vi "Init6733.vi"(8 "error in":errorcluster caption="错误输入") -> (0 "error out":errorcluster caption="错误输出", 3 "task out":refnum<k21> caption="任务输出")   [LabVIEW 2014]
uses:
  <vilib>/DAQmx/create/channels.llb/DAQmx Create Channel (AO-Voltage-Basic).vi
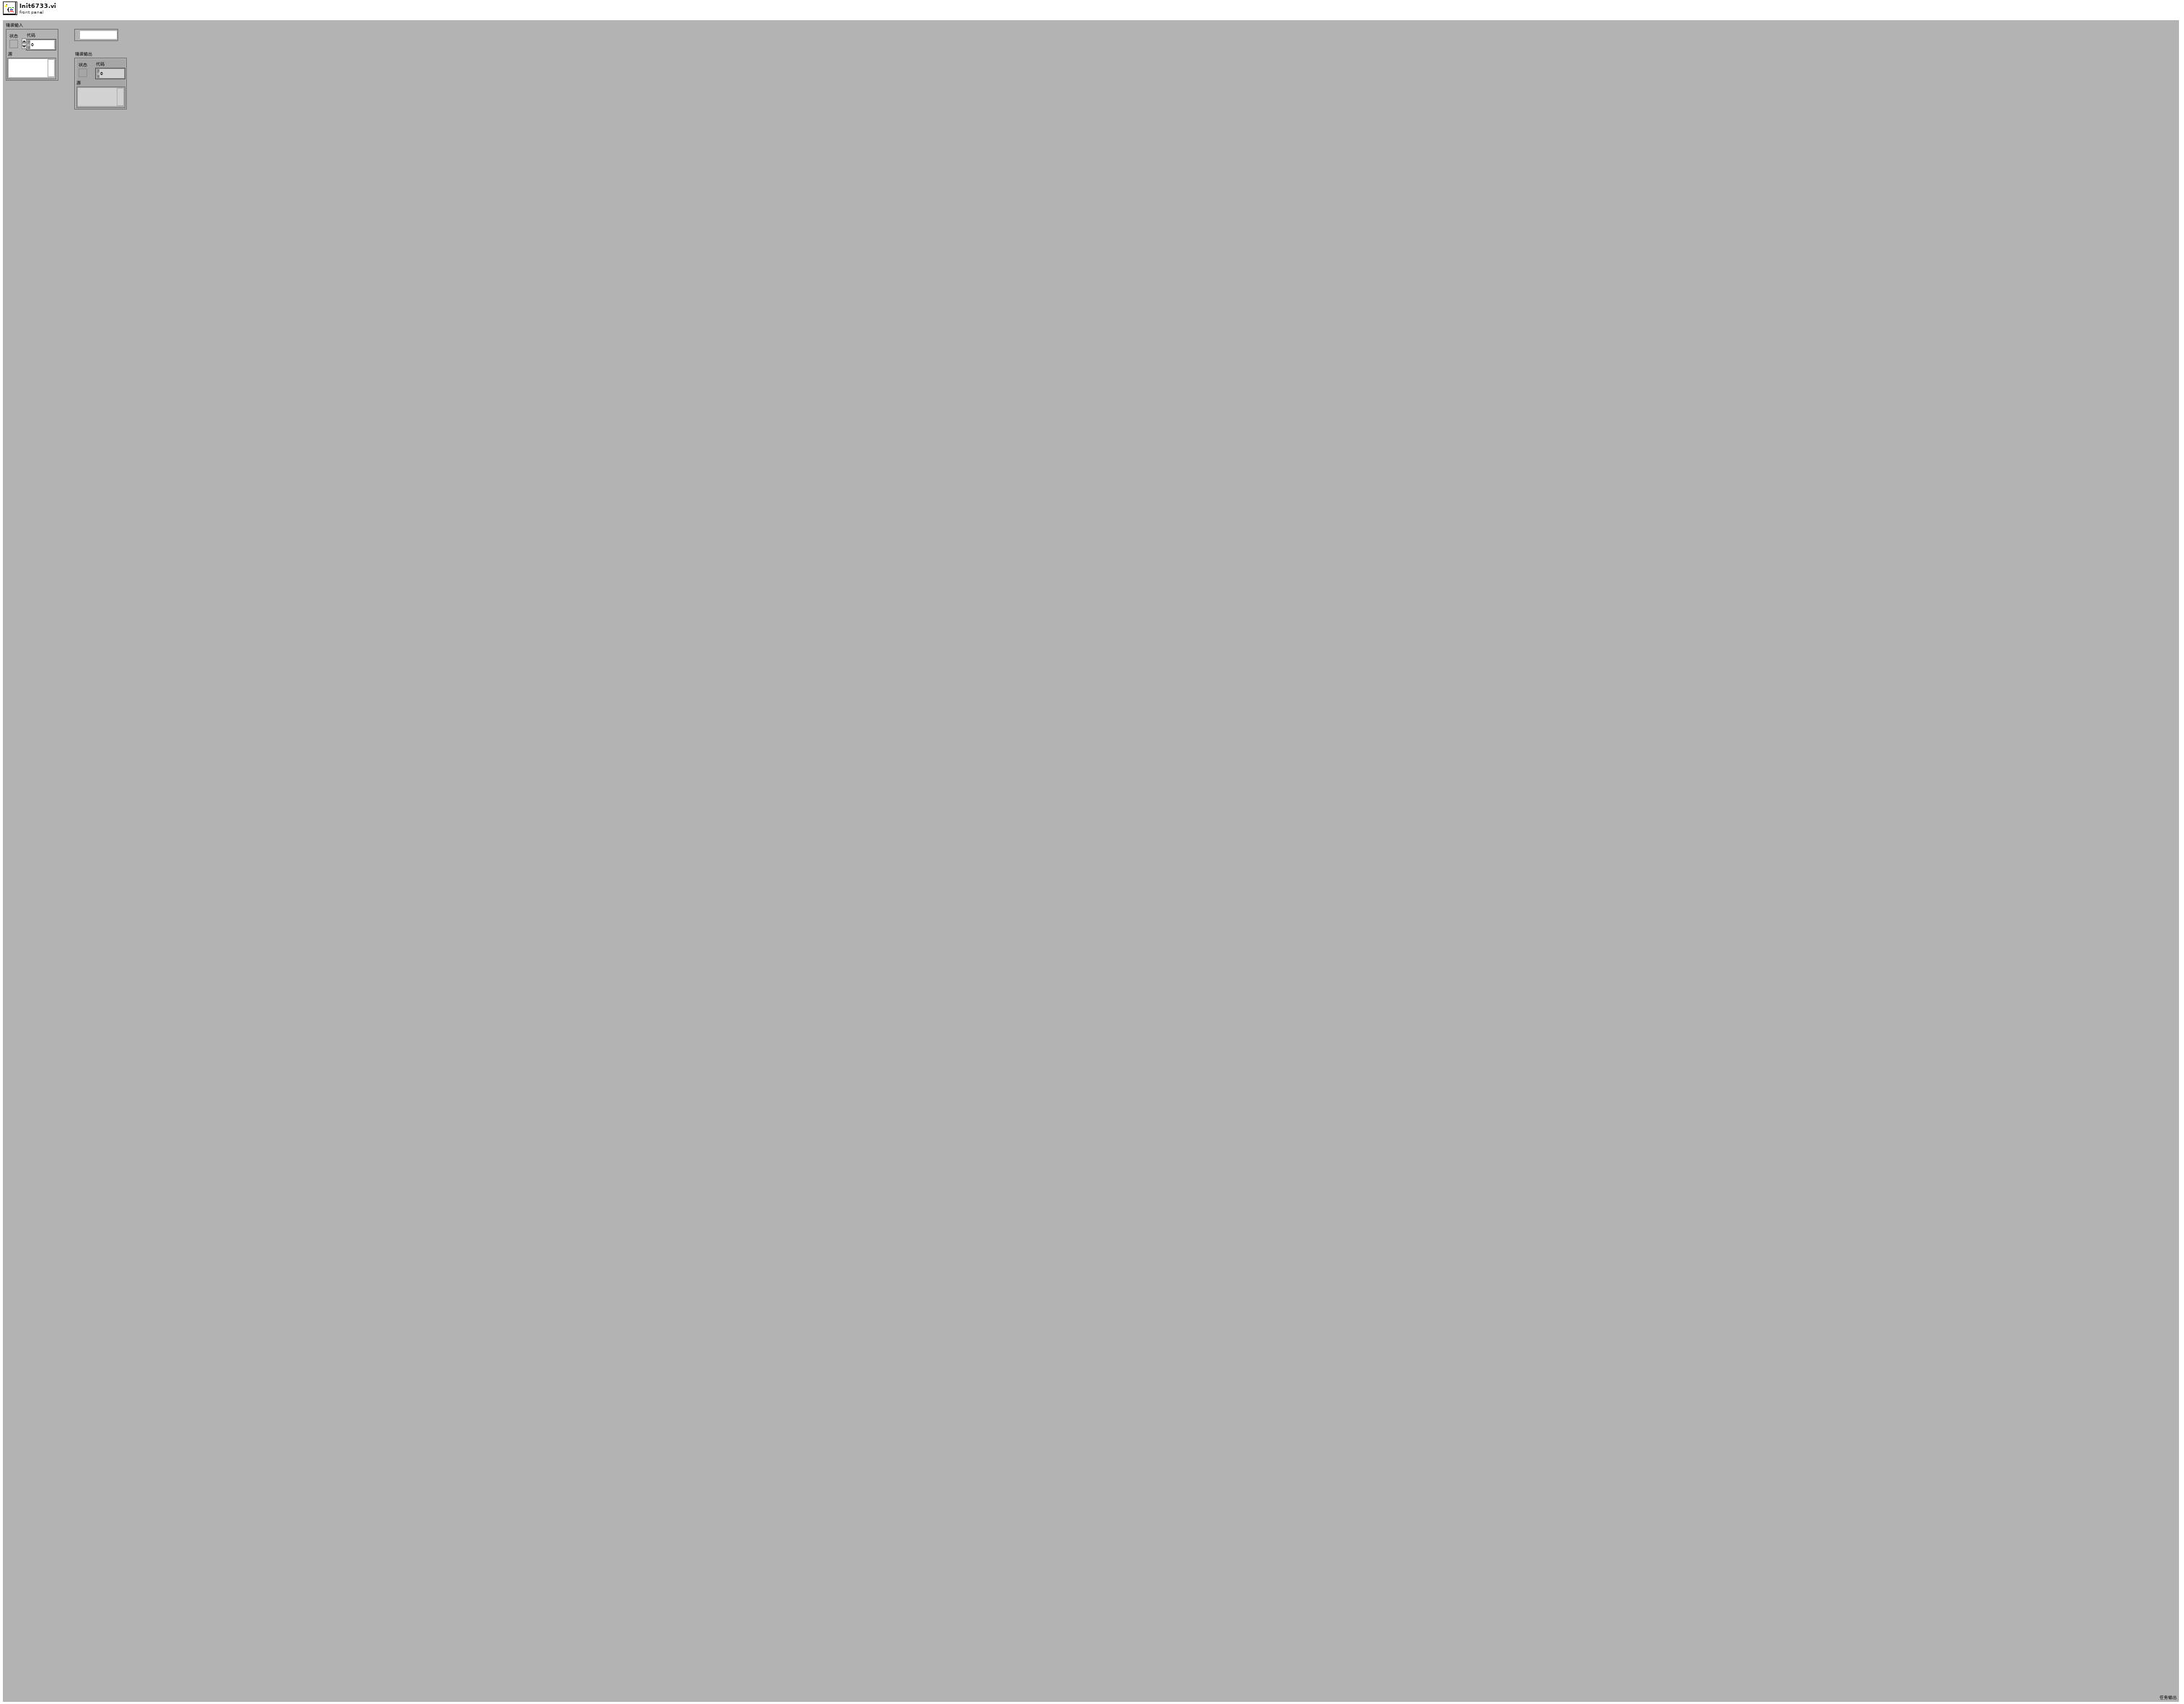
[diagram p1: front panel]
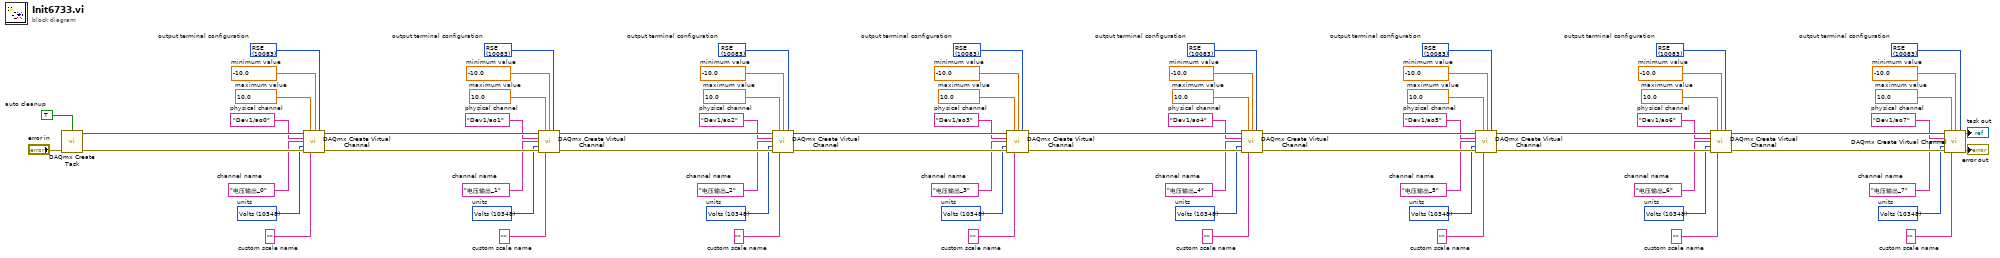
[diagram p0: block diagram]
diagram:
  w1 = 10083 items=["Default"=-1, "RSE"=10083, "Differential"=10106, "Pseudodifferential"=12529]  # output terminal configuration
  w2 = 10348 items=["Volts"=10348, "From Custom Scale"=10065]  # units
  w3 = "电压输出_7"  # channel name
  w6 = ""  # custom scale name
  w7 = -10.0  # minimum value
  w8 = 10.0  # maximum value
  w9 = "Dev1/ao7"  # physical channel
  w11 = 10083 items=["Default"=-1, "RSE"=10083, "Differential"=10106, "Pseudodifferential"=12529]  # output terminal configuration
  w12 = 10348 items=["Volts"=10348, "From Custom Scale"=10065]  # units
  w13 = "电压输出_6"  # channel name
  w15 = ""  # custom scale name
  w16 = -10.0  # minimum value
  w17 = 10.0  # maximum value
  w18 = "Dev1/ao6"  # physical channel
  w20 = 10083 items=["Default"=-1, "RSE"=10083, "Differential"=10106, "Pseudodifferential"=12529]  # output terminal configuration
  w21 = 10348 items=["Volts"=10348, "From Custom Scale"=10065]  # units
  w22 = "电压输出_5"  # channel name
  w24 = ""  # custom scale name
  w25 = -10.0  # minimum value
  w26 = 10.0  # maximum value
  w27 = "Dev1/ao5"  # physical channel
  w29 = 10083 items=["Default"=-1, "RSE"=10083, "Differential"=10106, "Pseudodifferential"=12529]  # output terminal configuration
  w30 = 10348 items=["Volts"=10348, "From Custom Scale"=10065]  # units
  w31 = "电压输出_4"  # channel name
  w33 = ""  # custom scale name
  w34 = -10.0  # minimum value
  w35 = 10.0  # maximum value
  w36 = "Dev1/ao4"  # physical channel
  w38 = 10083 items=["Default"=-1, "RSE"=10083, "Differential"=10106, "Pseudodifferential"=12529]  # output terminal configuration
  w39 = 10348 items=["Volts"=10348, "From Custom Scale"=10065]  # units
  w40 = "电压输出_3"  # channel name
  w42 = ""  # custom scale name
  w43 = -10.0  # minimum value
  w44 = 10.0  # maximum value
  w45 = "Dev1/ao3"  # physical channel
  w47 = 10083 items=["Default"=-1, "RSE"=10083, "Differential"=10106, "Pseudodifferential"=12529]  # output terminal configuration
  w48 = 10348 items=["Volts"=10348, "From Custom Scale"=10065]  # units
  w49 = "电压输出_2"  # channel name
  w51 = ""  # custom scale name
  w52 = -10.0  # minimum value
  w53 = 10.0  # maximum value
  w54 = "Dev1/ao2"  # physical channel
  w56 = 10083 items=["Default"=-1, "RSE"=10083, "Differential"=10106, "Pseudodifferential"=12529]  # output terminal configuration
  w57 = 10348 items=["Volts"=10348, "From Custom Scale"=10065]  # units
  w58 = "电压输出_1"  # channel name
  w60 = ""  # custom scale name
  w61 = -10.0  # minimum value
  w62 = 10.0  # maximum value
  w63 = "Dev1/ao1"  # physical channel
  w65 = 10083 items=["Default"=-1, "RSE"=10083, "Differential"=10106, "Pseudodifferential"=12529]  # output terminal configuration
  w66 = 10348 items=["Volts"=10348, "From Custom Scale"=10065]  # units
  w67 = "电压输出_0"  # channel name
  w69 = ""  # custom scale name
  w70 = -10.0  # minimum value
  w71 = 10.0  # maximum value
  w72 = "Dev1/ao0"  # physical channel
  w74 = TRUE  # auto cleanup
  n1 = call <vilib>:"DAQmx Create Task.vi"("auto cleanup"=w74, "error in"="error in") -> ("task out"=w73:refnum<k21>, "error out"=w75:errorcluster)  [unwired: 12 in]
  n2 = call-poly <vilib>:"DAQmx Create Virtual Channel.vi"("task in"=w73, "maximum value"=w71, "minimum value"=w70, "output terminal configuration"=w65, "physical channels"=w72, "name to assign"=w67, "units"=w66, "error in"=w75, "custom scale name"=w69) -> ("task out"=w64:refnum<k21>, "error out"=w68:errorcluster)  [unwired: 5 in]
  n3 = call-poly <vilib>:"DAQmx Create Virtual Channel.vi"("task in"=w64, "maximum value"=w62, "minimum value"=w61, "output terminal configuration"=w56, "physical channels"=w63, "name to assign"=w58, "units"=w57, "error in"=w68, "custom scale name"=w60) -> ("task out"=w55:refnum<k21>, "error out"=w59:errorcluster)  [unwired: 5 in]
  n4 = call-poly <vilib>:"DAQmx Create Virtual Channel.vi"("task in"=w55, "maximum value"=w53, "minimum value"=w52, "output terminal configuration"=w47, "physical channels"=w54, "name to assign"=w49, "units"=w48, "error in"=w59, "custom scale name"=w51) -> ("task out"=w46:refnum<k21>, "error out"=w50:errorcluster)  [unwired: 5 in]
  n5 = call-poly <vilib>:"DAQmx Create Virtual Channel.vi"("task in"=w46, "maximum value"=w44, "minimum value"=w43, "output terminal configuration"=w38, "physical channels"=w45, "name to assign"=w40, "units"=w39, "error in"=w50, "custom scale name"=w42) -> ("task out"=w37:refnum<k21>, "error out"=w41:errorcluster)  [unwired: 5 in]
  n6 = call-poly <vilib>:"DAQmx Create Virtual Channel.vi"("task in"=w37, "maximum value"=w35, "minimum value"=w34, "output terminal configuration"=w29, "physical channels"=w36, "name to assign"=w31, "units"=w30, "error in"=w41, "custom scale name"=w33) -> ("task out"=w28:refnum<k21>, "error out"=w32:errorcluster)  [unwired: 5 in]
  n7 = call-poly <vilib>:"DAQmx Create Virtual Channel.vi"("task in"=w28, "maximum value"=w26, "minimum value"=w25, "output terminal configuration"=w20, "physical channels"=w27, "name to assign"=w22, "units"=w21, "error in"=w32, "custom scale name"=w24) -> ("task out"=w19:refnum<k21>, "error out"=w23:errorcluster)  [unwired: 5 in]
  n8 = call-poly <vilib>:"DAQmx Create Virtual Channel.vi"("task in"=w19, "maximum value"=w17, "minimum value"=w16, "output terminal configuration"=w11, "physical channels"=w18, "name to assign"=w13, "units"=w12, "error in"=w23, "custom scale name"=w15) -> ("task out"=w10:refnum<k21>, "error out"=w14:errorcluster)  [unwired: 5 in]
  n9 = call-poly <vilib>:"DAQmx Create Virtual Channel.vi"("task in"=w10, "maximum value"=w8, "minimum value"=w7, "output terminal configuration"=w1, "physical channels"=w9, "name to assign"=w3, "units"=w2, "error in"=w14, "custom scale name"=w6) -> ("task out"=→"task out":refnum<k21>, "error out"=→"error out":errorcluster)  [unwired: 5 in]
